vi "CRYResample Compute Padding Zeros.vi"(4 "padding zeros?":bool=TRUE, 5 "anti-aliasing?":bool=TRUE, 6 "FIR filter specifications":T1={"alias rejection (dB)"=120.0, "normalized bandwidth"=0.4536} {"normalized bandwidth" format="%.4f"; "alias rejection (dB)" format="%.2f"}, 7 "reset?":bool, 8 "error in (no error)":errorcluster, 9 "dt":dbl=1.0, 10 "delay":dbl, 11 "X":dbl[](array[numeric])) -> (0 "error out":errorcluster, 2 "length of Y":i32, 3 "length of padding zeros":i32)   [LabVIEW 2013]
doc: "Determine the length of padding zeroes needed in order to get the resampled signal of the same time span as the input signal <B>X</B>."
uses:
  <vilib>/Analysis/NI_AALPro.lvlib
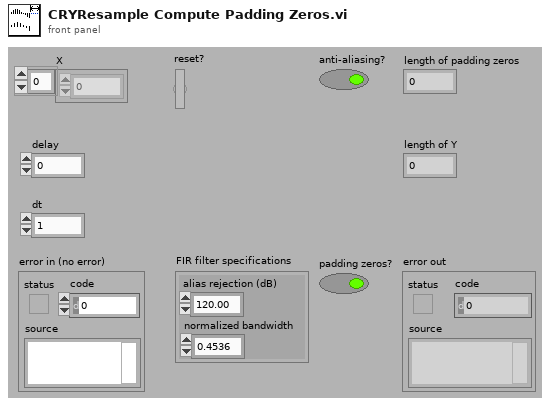
[diagram p1: front panel]
types:
  T1 = cluster{"alias rejection (dB)":dbl, "normalized bandwidth":dbl}
  T2 = cluster{"new sample period":dbl, "Timing Jitter":enum32{"Interpolation", "Rounding"}, "first point location":dbl, "prototype filter":cluster{"h":dbl[], "Max Decimation":i32}}
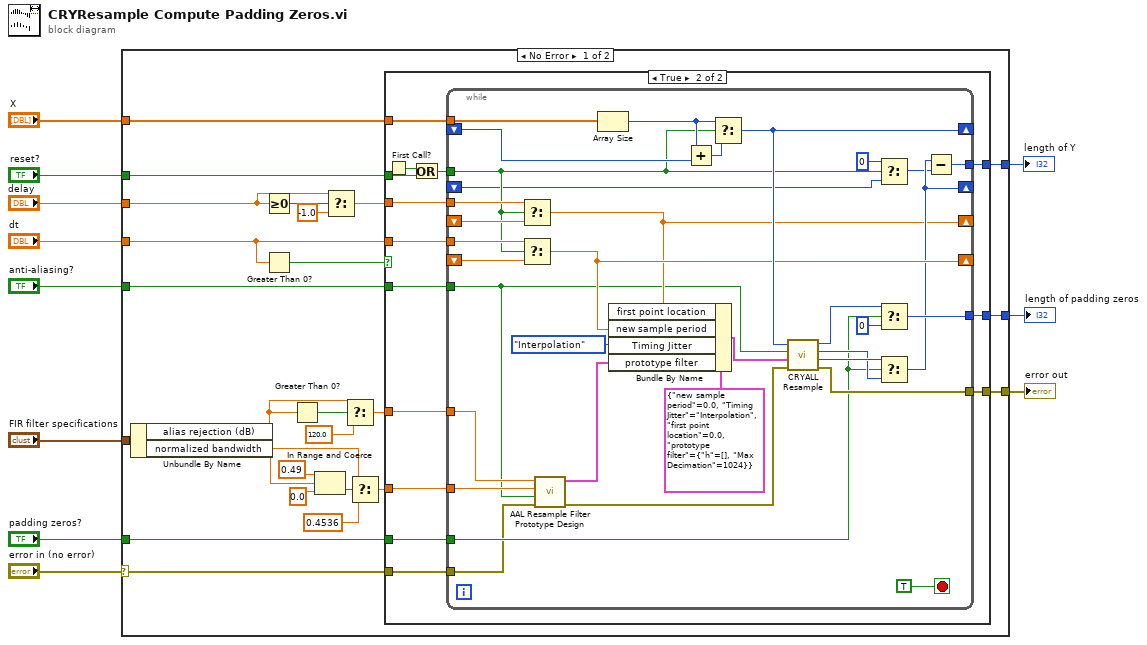
[diagram p0: block diagram]
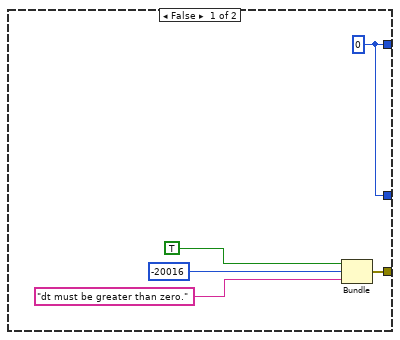
[diagram p2: hidden frame]
diagram:
  n1 = case shown="No Error" "error in (no error)" {
    selector: "error in (no error)" -> [w13 w90]
    tunnel: [w36 w90] -> w11
    tunnel: "dt" -> [w34 _]
    tunnel: "FIR filter specifications" -> [w33 _]
    tunnel: "reset?" -> [w22 _]
    tunnel: "delay" -> [w20 _]
    tunnel: [w17 _] -> w6
    tunnel: "anti-aliasing?" -> [w16 _]
    tunnel: "X" -> [w15 _]
    tunnel: "padding zeros?" -> [w14 _]
    tunnel: [w12 _] -> w1
    frame No Error {
      n2 = Unbundle By Name(w33) -> ("alias rejection (dB)"=w23:dbl, "normalized bandwidth"=w27:dbl)
      n3 = Greater Or Equal To 0?(x=w20) -> (x >= 0?=w21:bool)
      n4 = Greater Than 0?(x=w34) -> (x > 0?=w35:bool)
      n5 = Greater Than 0?(x=w23) -> (x > 0?=w24:bool)
      n6 = In Range and Coerce(upper limit=0.49, x=w27, lower limit=0.0 ("upper limit")) -> (In Range?=w28:bool)  [unwired: 1 out]
      n7 = Select(t=w20, s=w21, f=-1.0) -> (s? t:f=w18:dbl)
      n8 = Select(t=w23, s=w24, f=120.0) -> (s? t:f=w29:dbl)
      n9 = Select(t=w27, s=w28, f=0.4536 ("upper limit")) -> (s? t:f=w25:dbl)
      n10 = case shown="True" w35 {
        tunnel: w18 -> [_ w47]
        tunnel: [w41 w55] -> w36
        tunnel: w34 -> [_ w54]
        tunnel: w29 -> [_ w53]
        tunnel: w25 -> [_ w52]
        tunnel: w22 -> [_ w50]
        tunnel: [w37 w48] -> w17
        tunnel: w16 -> [_ w46]
        tunnel: w15 -> [_ w45]
        tunnel: w14 -> [_ w44]
        tunnel: w13 -> [_ w43]
        tunnel: [w37 w42] -> w12
        frame False {
          w37 = 0 ("length of padding zeroes")
          n11 = Bundle(TRUE, "DtGTZeroErr"=-20016, "dt must be greater than zero.") -> (w41:cluster{bool, "DtGTZeroErr":i32, string})  [unwired: 1 in]
        }
        frame True {
          n12 = First Call?() -> (First Call?: T/F=w51:bool)
          n13 = Or(x=w51, y=w50) -> (x .or. y?=w49:bool)
          n14 = while {
            tunnel: [w89] -> w55
            tunnel: w54 -> [w76]
            tunnel: w53 -> [w88]
            tunnel: w52 -> [w87]
            tunnel: [w73] -> w42
            tunnel: w49 -> [w65]
            shift-right: [w79] -> _
            shift-left: _ -> [w80]
            tunnel: [w70] -> w48
            shift-right: [w74] -> _
            shift-left: _ -> [w75]
            shift-right: [w69] -> _
            shift-left: _ -> [w62]
            shift-right: [w66] -> _
            shift-left: _ -> [w68]
            tunnel: w47 -> [w67]
            tunnel: w46 -> [w59]
            tunnel: w45 -> [w58]
            tunnel: w44 -> [w57]
            tunnel: w43 -> [w56]
            stop <- TRUE stop-if-true
            n15 = Select(t=w67, s=w65, f=w68) -> (s? t:f=w66:dbl)
            n16 = Select(t=w76, s=w65, f=w75) -> (s? t:f=w74:dbl)
            n17 = call <vilib>:"AAL Resample Filter Prototype Design.vi"("error in (no error)"=w56, "alias free"=w59, "normalized bandwidth"=w87, "A stop [dB]"=w88) -> ("error out"=w83:errorcluster, "filter prototype"=w84:cluster{"coefficients":dbl[], "factor":i32})  [unwired: 5 in, 1 out]
            n18 = Array Size(array=w58) -> (size(s)=w81:i32)
            n19 = Bundle By Name(cluster=T2 {"new sample period"=0.0, "Timing Jitter"=enum."Interpolation", "first point location"=0.0, "prototype filter"={"h"=[], "Max Decimation"=1024}} ("config"), "first point location"=w66, "new sample period"=w74, "Timing Jitter"=enum32{"Interpolation", "Rounding"}."Interpolation" ("timing jitter"), "prototype filter"=w84) -> (w77:T2)
            n20 = Add(x=w81, y=w80) -> (x+y=w82:i32)
            n21 = Select(t=w81, s=w65, f=w82) -> (s? t:f=w79:i32)
            n22 = call "CRYALL Resample.vi"("error in (no error)"=w83, "config"=w77, "anti-aliasing?"=w59, "length of X"=w79) -> ("error out"=w89:errorcluster, "length of Y (after padding zeroes)"=w61:i32, "length of Y"=w60:i32, "length of padding zeroes"=w72:i32)  [unwired: 4 in]
            n23 = Select(t=0, s=w65, f=w62) -> (s? t:f=w64:i32)
            n24 = Select(t=w72, s=w57, f=0) -> (s? t:f=w73:i32)
            n25 = Select(t=w61, s=w57, f=w60) -> (s? t:f=w69:i32)
            n26 = Subtract(x=w69, y=w64) -> (x-y=w70:i32)
          }
        }
      }
    }
    frame Error {
    }
  }
  "error out" <- w11
  "length of padding zeros" <- w1
  "length of Y" <- w6
